vi "Read_Redudant.vi"(0 ".NET Refnum in":refnum<k24>, 1 "Read ERD List In":T2[](array[typedef]) {"ERD Number" format="%.0x"}, 3 "GEA Inputs":T4 {"Destination" format="%.0x"; "Source" format="%.0x"}, 5 "error in (no error)":errorcluster) -> (14 ".NET Refnum out":refnum<k24>, 15 "Read ERD List Out":T2[](array[typedef]) {"ERD Number" format="%.0x"}, 16 "ERD Data Out":T1[](array[typedef]) {"ERD Number" format="%.0x"}, 17 "F011 not Present":bool, 19 "error out":errorcluster)   [LabVIEW 2016]
doc: "This VI checks to see if Accelerometer ERD is in Read ERD List. If so it write to Accelerometer ERD. Writing toi this ERD updates ERD with latest Accelerometer data, which allows it to be read back from ERD."
uses:
  Common/LabVIEW GEA2 Toolkit/LabVIEW_GEA2_Toolkit.lvlibp/type defs/ERD Read Data In.ctl
  Common/LabVIEW GEA2 Toolkit/LabVIEW_GEA2_Toolkit.lvlibp/type defs/Data Type.ctl
  Common/LabVIEW GEA2 Toolkit/LabVIEW_GEA2_Toolkit.lvlibp/type defs/Source_Destination.ctl
  C:/Automation/DLLs/PC Dot Net/GeaCommunication.dll
  Common/LabVIEW GEA2 Toolkit/LabVIEW_GEA2_Toolkit.lvlibp/type defs/ERD Read Data Out.ctl
  Common/LabVIEW GEA2 Toolkit/LabVIEW_GEA2_Toolkit.lvlibp
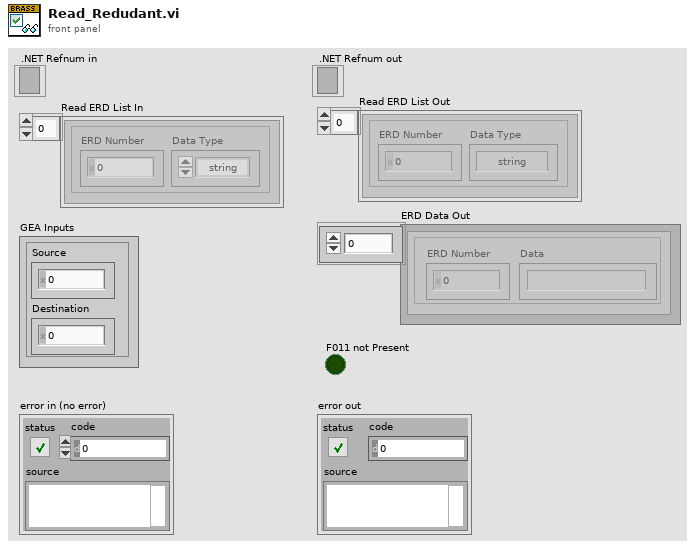
[diagram p1: front panel]
types:
  T1 = typedef "LabVIEW_GEA2_Toolkit.lvlibp/ERD Read Data Out.ctl" = cluster{"ERD Number":u16, "Data":string}
  T2 = typedef "LabVIEW_GEA2_Toolkit.lvlibp/ERD Read Data In.ctl" = cluster{"ERD Number":u16, "Data Type":T3}
  T3 = typedef "LabVIEW_GEA2_Toolkit.lvlibp/Data Type.ctl" = enum16{"string", "boolean", "uint8_t", "uint16_t", "uint32_t", "uint64_t", "int8_t", "int16_t", "int32_t", "int64_t"}
  T4 = typedef "LabVIEW_GEA2_Toolkit.lvlibp/Source_Destination.ctl" = cluster{"Source":u8, "Destination":u8}
  T5 = typedef "LabVIEW_GEA2_Toolkit.lvlibp/Data In.ctl" = cluster{"Source":u8, "Destination":u8, "Command":u8, "Message":string}
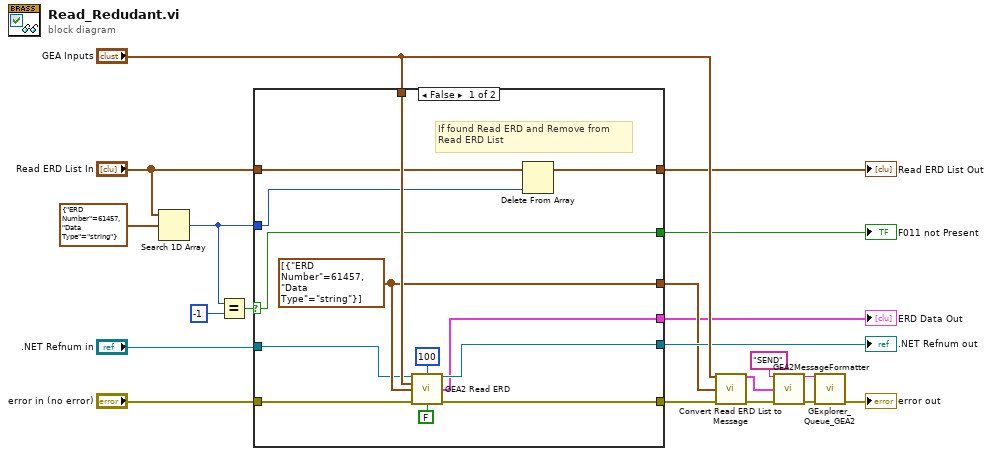
[diagram p0: block diagram]
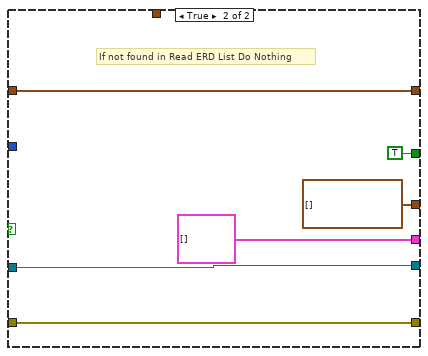
[diagram p2: hidden frame]
diagram:
  n1 = Search 1D Array(1D array="Read ERD List In", element=T2 {"ERD Number"=61457, "Data Type"=enum."string"}) -> (index of element=w5:i32)  [unwired: 1 in]
  n2 = Equal?(x=w5, y=-1) -> (x = y?=w19:bool)
  n3 = case shown="False" w19 {
    selector: w19 -> [w21 _]
    tunnel: "error in (no error)" -> [w31 w38]
    tunnel: [w30 w38] -> w10
    tunnel: ".NET Refnum in" -> [w22 w39]
    tunnel: [w24 w39] -> w7
    tunnel: "GEA Inputs" -> [w29 _]
    tunnel: [w28 T2[] [] ("Read ERD List")] -> w6
    tunnel: w5 -> [w26 _]
    tunnel: "Read ERD List In" -> [w27 w36]
    tunnel: [w25 w36] -> w3
    tunnel: [w23 T1[] [] ("ERD Data Out")] -> w2
    tunnel: [w21 TRUE] -> w1
    frame False {
      w28 = T2[] [{"ERD Number"=61457, "Data Type"=enum."string"}] ("Read ERD List")
      # "If found Read ERD and Remove from\nRead ERD List"
      n4 = call "GEA2 Read ERD.vi"("GEA2 Reference In"=w22, "Read Timeout (ms)"=u32 100, "GEA Inputs"=w29, "Read ERD List"=w28, "Error In"=w31, "Verify ERD Response?"=FALSE) -> ("GEA2 Reference Out"=w24:refnum<k24>, "ERD Data Out"=w23:T1[], "Error Out"=w30:errorcluster)  [unwired: 6 in, 1 out]
      n5 = Delete From Array(array=w27, index=w26) -> (array with subset deleted=w25:T2[])  [unwired: 1 in, 1 out]
    }
    frame True {
      # "If not found in Read ERD List Do Nothing"
    }
  }
  ".NET Refnum out" <- w7
  "Read ERD List Out" <- w3
  "ERD Data Out" <- w2
  "F011 not Present" <- w1
  n6 = call "Convert Read ERD List to Message.vi"("GEA Inputs"="GEA Inputs", "Read ERD List"=w6, "Error In"=w10) -> ("GEA Message"=w14:T5, "Error Out"=w15:errorcluster)  [unwired: 11 in]
  n7 = call "GEA2MessageFormatter.vi"("Prefix(Send/Recv)"="SEND", "GEA2 Data In"=w14, "Error In"=w15) -> ("Output String"=w13:string, "Error Out"=w12:errorcluster)  [unwired: 11 in]
  n8 = call "GExplorer_Queue_GEA2.vi"("Output String"=w13, "error in (no error)"=w12) -> ("error out"=→"error out":errorcluster)  [unwired: 13 in]
